vi "osc_scope_to_word.vi"() -> ()   [LabVIEW 2026]
uses:
  <vilib>/Utility/NIReport.llb/Report Type.ctl
  <vilib>/Utility/NIReport.llb/Append Text Table to Report (wrap).vi
  <vilib>/Utility/NIReport.llb/NI_report.lvclass
  <vilib>/wsapi/NI_WebServices.lvlib
  <vilib>/Utility/NIReport.llb/NI_ReportGenerationCore.lvlib
panel:
  out "error out":errorcluster
  in  "device table":string[][](array[string])=[["dede", ""], ["", "ddddd"]]
  out "2D Picture 2":picture
  in  "write buffer":string=":DISPlay:DATA? PNG, COLOR"
  in  "VISA resource name":refnum<visa-resource-name>
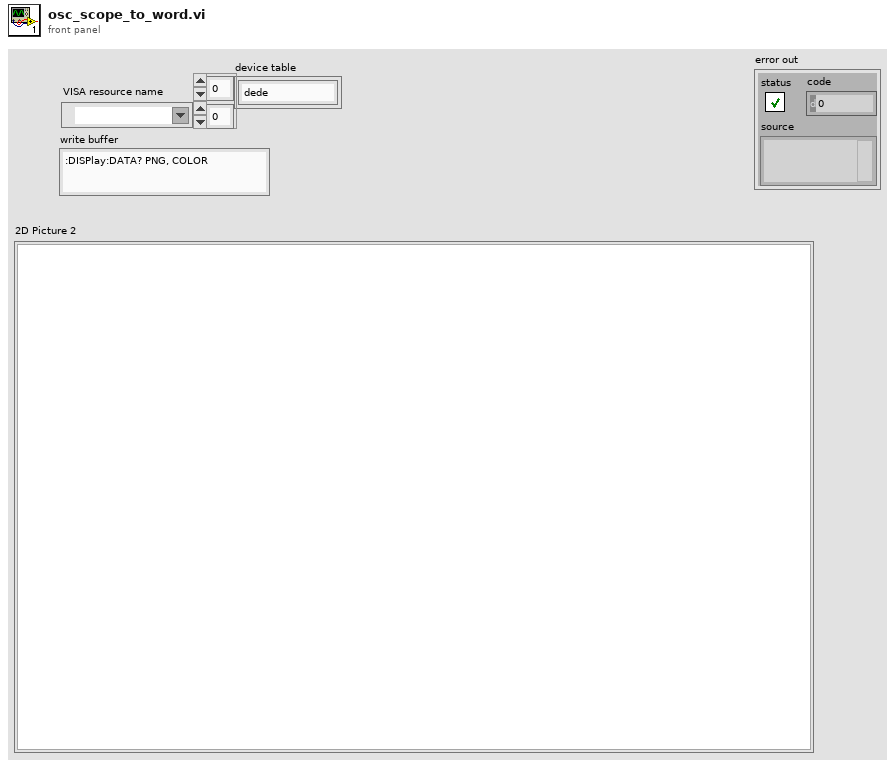
[diagram p1: front panel]
types:
  T1 = typedef "NI_ReportGenerationCore.lvlib/Report Type.ctl" = enum16{"HTML", "Word", "Excel"}
  T2 = typedef "imagedata.ctl" = cluster{"image type":i32, "image depth":i32, "image":u8[], "mask":u8[], "colors":u32[], "Rectangle":cluster{"left":i16, "top":i16, "right":i16, "bottom":i16}}
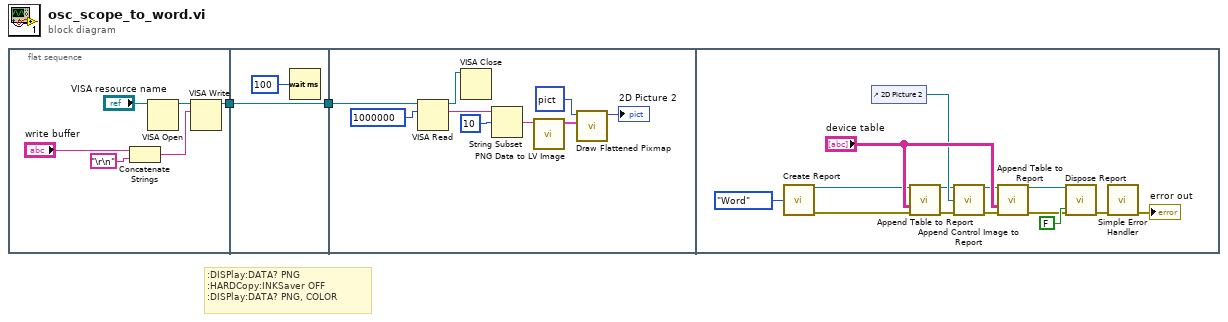
[diagram p0: block diagram]
diagram:
  # ":DISPlay:DATA? PNG\n:HARDCopy:INKSaver OFF\n:DISPlay:DATA? PNG, COLOR"
  n1 = flat-sequence {
    tunnel: [w3] -> w2
    tunnel: w2 -> [w9]
    tunnel: [w9] -> w1
    tunnel: w1 -> [w18]
    frame #0 {
      n2 = Concatenate Strings("write buffer", "\r\n") -> (w4:string)
      n3 = VISA Open(VISA resource name="VISA resource name") -> (VISA resource name=w7:refnum<visa-resource-name>)  [unwired: 4 in, 1 out]
      n4 = VISA Write(VISA resource name=w7, write buffer=w4) -> (VISA resource name out=w3:refnum<visa-resource-name>)  [unwired: 1 in, 2 out]
    }
    frame #1 {
      n5 = Wait (ms)(milliseconds to wait=u32 100) -> ()  [unwired: 1 out]
    }
    frame #2 {
      n6 = VISA Read(VISA resource name=w18, byte count=u32 1000000) -> (VISA resource name out=w13:refnum<visa-resource-name>, read buffer=w14:string)  [unwired: 1 in, 2 out]
      n7 = VISA Close(VISA resource name=w13) -> ()  [unwired: 1 in, 1 out]
      n8 = String Subset(string=w14, offset (0)=10) -> (substring=w17:string)  [unwired: 1 in]
      n9 = call <vilib>:"PNG Data to LV Image.vi"("png data"=w17) -> ("image data"=w11:T2)  [unwired: 9 in, 1 out]
      n10 = call <vilib>:"Draw Flattened Pixmap.vi"("image data"=w11, "picture"=picture data[5B]) -> ("new picture"=→"2D Picture 2":picture)  [unwired: 7 in]
    }
    frame #3 {
      n11 = call <vilib>:"Create Report.vi"("report type"=Report_Type."Word" ("Report Type")) -> ("report out"=w27:refnum<class "NI_report.lvclass">, "error out"=w26:errorcluster)  [unwired: 13 in]
      n12 = control-ref of="2D Picture 2"() -> (w29:refnum<vi>)
      n13 = call-poly <vilib>:"Append Table to Report.vi"("report in"=w27, "text data"="device table", "error in (no error)"=w26) -> ("report out"=w28:refnum<class "NI_report.lvclass">, "error out"=w33:errorcluster)  [unwired: 9 in, 2 out]
      n14 = call-dynamic "Append Control Image to Report.vi"("report in"=w28, "ctrl reference"=w29, "error in (no error)"=w33) -> ("report out"=w30:refnum<class "NI_report.lvclass">, "error out"=w32:errorcluster)  [unwired: 9 in, 2 out]
      n15 = call-poly <vilib>:"Append Table to Report.vi"("report in"=w30, "text data"="device table", "error in (no error)"=w32) -> ("report out"=w21:refnum<class "NI_report.lvclass">, "error out"=w20:errorcluster)  [unwired: 9 in, 2 out]
      n16 = call-dynamic "Dispose Report.vi"("report in"=w21, "error in (no error)"=w20, "close report? (T)"=FALSE ("Close Report? (T)")) -> ("error out"=w23:errorcluster)  [unwired: 12 in]
      n17 = call <vilib>:"Simple Error Handler.vi"("error in (no error)"=w23) -> ("error out"=→"error out":errorcluster)  [unwired: 4 in, 4 out]
    }
  }
